vi "panel2.vi"(8 "error in (no error)":errorcluster) -> (0 "error out":errorcluster)   [LabVIEW 2017]
uses:
  a288a1d7-2791-4915-a0b1-330fddf74d70.vi
  0919d1f0-e5d2-482b-8841-45466cc748b4.vi
  TagDB/_Support/DataAccess/_NameCacher.vi
  TagDB/_Support/DataAccess/TagDB Ref to DVR.vi
  <vilib>/Utility/error.llb/Trim Whitespace.vi
  TagDB/_Support/Error/_[error50000]Invalid DB REF.vi
  TagDB/_Support/Error/_[error50002]Invalid DataType.vi
  TagDB/TagDB(DEV).lvlib
panel:
  out "value 2":variant
  out "Test send message":string
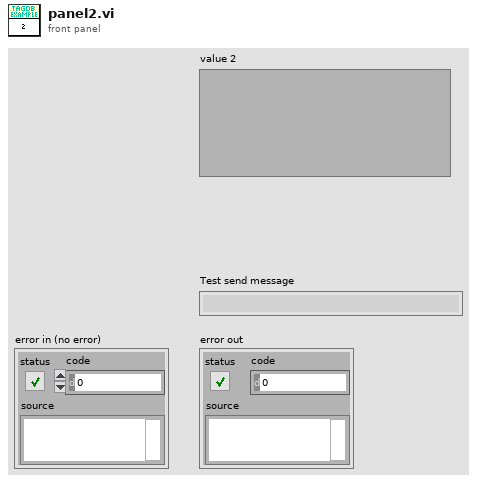
[diagram p1: front panel]
types:
  T1 = typedef "TagDB(DEV).lvlib/TagContainer.ctl" = refnum<k1>
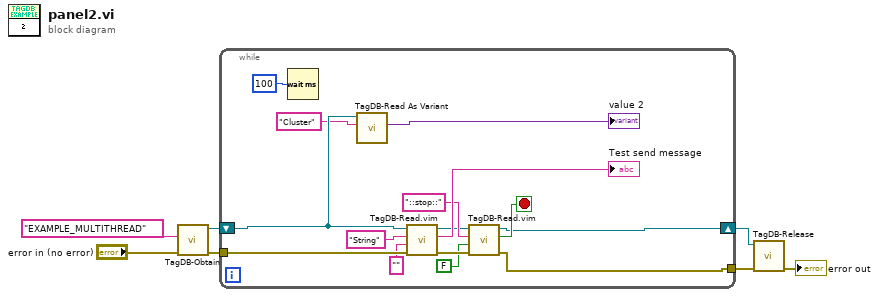
[diagram p0: block diagram]
diagram:
  n1 = call "TagDB-Obtain.vi"("error in (no error)"="error in (no error)", "name (unnamed)"="EXAMPLE_MULTITHREAD") -> ("error out"=w5:errorcluster, "TagContainer"=w4:T1)  [unwired: 3 in, 1 out]
  n2 = while {
    tunnel: w5 -> [w20]
    tunnel: [w13] -> w6
    shift-right: [w14] -> w1
    shift-left: w4 -> [w12]
    stop <- w18 stop-if-true
    n3 = Wait (ms)(milliseconds to wait=u32 100) -> ()  [unwired: 1 out]
    n4 = call "TagDB-Read As Variant.vi"("name"="Cluster", "TagContainer"=w12) -> ("Value"=→"value 2":variant)  [unwired: 4 in, 5 out]
    n5 = call "TagDB-Read.vim"("error in (no error)"=w20, "Type"="", "name"="String", "TagContainer"=w12) -> ("error out"=w15:errorcluster, "Value"=→"Test send message":string, "TagContainer(dup)"=w16:T1)  [unwired: 2 in, 3 out]
    n6 = call "TagDB-Read.vim"("error in (no error)"=w15, "Type"=FALSE, "name"="::stop::", "TagContainer"=w16) -> ("error out"=w13:errorcluster, "Value"=w18:bool, "TagContainer(dup)"=w14:T1)  [unwired: 2 in, 3 out]
  }
  n7 = call "TagDB-Release.vi"("error in (no error)"=w6, "TagContainer"=w1) -> ("error out"=→"error out":errorcluster)  [unwired: 9 in]
